vi "FindVertexOrder.vi"(5 "order":T1(ring)=enum."reverse postorder", 9 "DAG in":refnum<class "DAG.lvclass">) -> (4 "vertices":i32[](array[numeric]))   [LabVIEW 2014, in "Raspberry Pi Compatible Compiler for LabVIEW.lvlib" / "DAG.lvclass"]
uses:
  DAG.lvclass
  TypeDefs/TraversalEnum.ctl
  DAG.lvclass/DAG.ctl
  Raspberry Pi Compatible Compiler for LabVIEW.lvlib
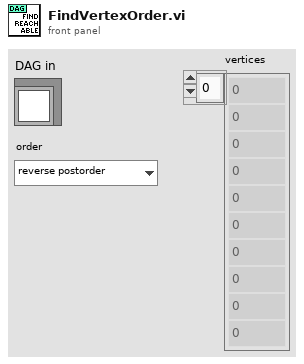
[diagram p1: front panel]
types:
  T1 = enum16{"preorder", "postorder", "reverse postorder"}
  T2 = typedef "Raspberry Pi Compatible Compiler for LabVIEW.lvlib/TraversalEnum.ctl" = enum16{"dfs", "pre-enqueue", "post-enqueue"}
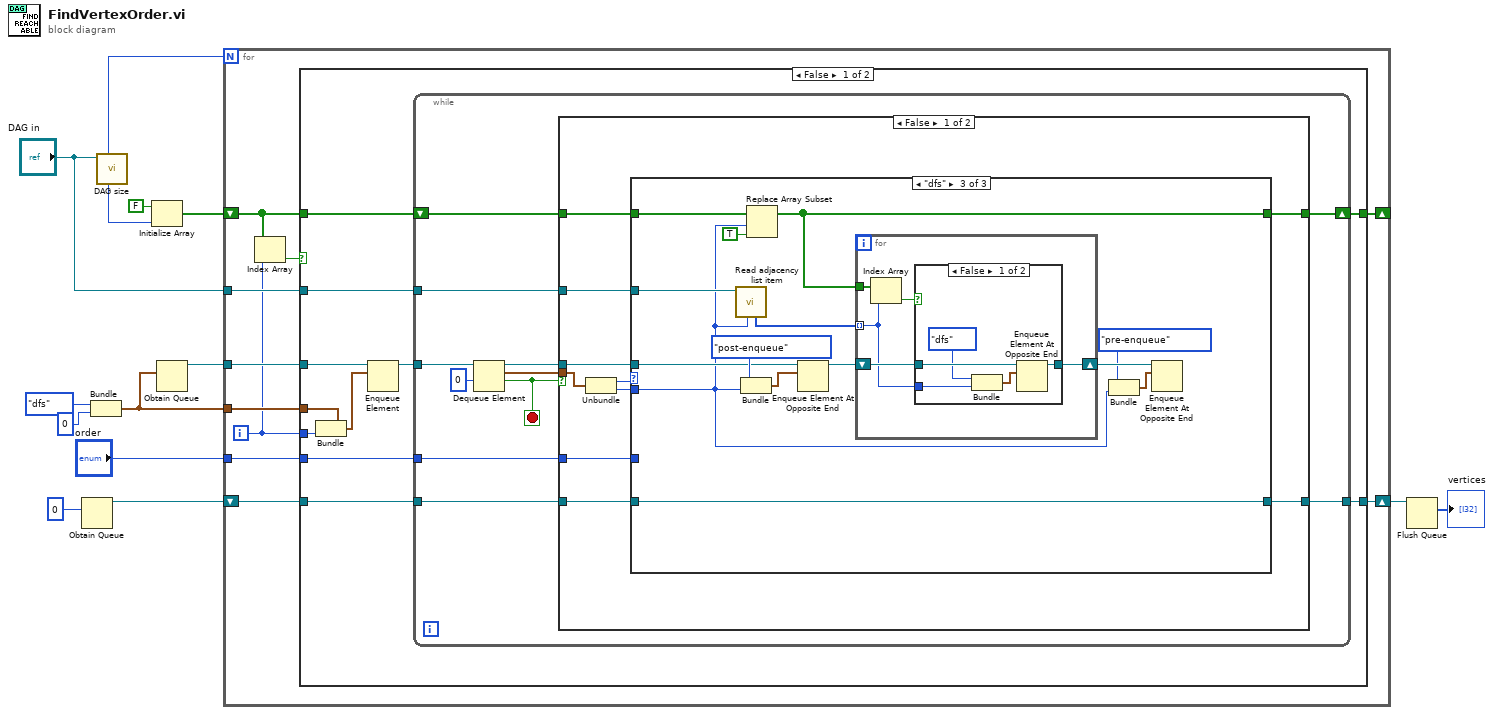
[diagram p0: block diagram]
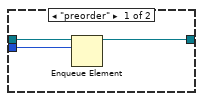
[diagram p3: hidden frame]
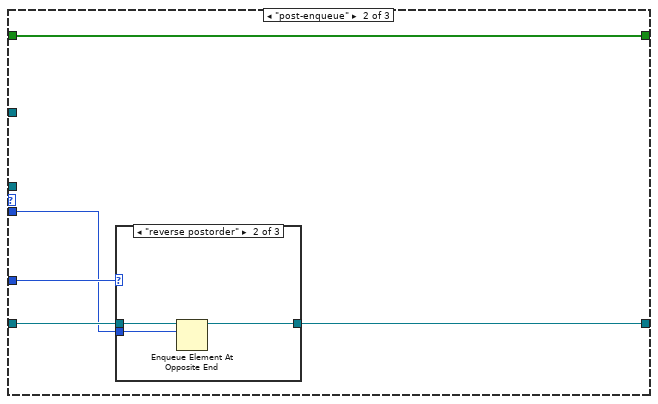
[diagram p4: hidden frame]
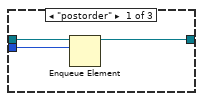
[diagram p5: hidden frame]
diagram:
  n1 = Obtain Queue(element data type=0 ("element")) -> (queue out=w5:refnum<queue>)  [unwired: 4 in, 2 out]
  n2 = Bundle(TraversalEnum."dfs", "element"=0) -> (w2:cluster{T2, "element":i32})  [unwired: 1 in]
  n3 = call "DAG size.vi"("DAG in"="DAG in") -> ("vertices"=w1:i32)  [unwired: 6 in, 2 out]
  n4 = Initialize Array(FALSE, w1) -> (w9:bool[])
  n5 = Obtain Queue(element data type=w2) -> (queue out=w10:refnum<queue>)  [unwired: 4 in, 2 out]
  n6 = for {
    N: w1 -> [_]
    tunnel: "DAG in" -> [w23]
    tunnel: w10 -> [w22]
    tunnel: "order" -> [w20]
    tunnel: w2 -> [w18]
    shift-right: [w17] -> _
    shift-left: w9 -> [w16]
    shift-right: [w19] -> w3
    shift-left: w5 -> [w21]
    i -> [w15]
    n7 = Index Array(array=w16, index=w15) -> (element=w14:bool)
    n8 = case shown="False" w14 {
      tunnel: w23 -> [w34 _]
      tunnel: w22 -> [w33 _]
      tunnel: w21 -> [w31 w104]
      tunnel: w20 -> [w30 _]
      tunnel: [w29 w104] -> w19
      tunnel: w18 -> [w28 _]
      tunnel: [w26 w105] -> w17
      tunnel: w16 -> [w25 w105]
      tunnel: w15 -> [w24 _]
      frame False {
        n9 = Bundle(cluster=w28, "element"=w24) -> (w27:cluster{T2, "element":i32})  [unwired: 1 in]
        n10 = Enqueue Element(queue=w33, element=w27) -> (queue out=w32:refnum<queue>)  [unwired: 2 in, 2 out]
        n11 = while {
          shift-right: [w42] -> w26
          shift-left: w25 -> [w41]
          tunnel: w32 -> [w45]
          tunnel: w34 -> [w40]
          tunnel: w31 -> [w37]
          tunnel: [w36] -> w29
          tunnel: w30 -> [w35]
          stop <- w43 stop-if-true
          n12 = Dequeue Element(queue=w45, timeout in ms (-1)=0) -> (queue out=w39:refnum<queue>, element=w38:cluster{T2, "element":i32}, timed out?=w43:bool)  [unwired: 1 in, 1 out]
          n13 = case shown="False" w43 {
            tunnel: w39 -> [w55 _]
            tunnel: [w53 w103] -> w42
            tunnel: w41 -> [w46 w103]
            tunnel: w38 -> [w52 _]
            tunnel: w40 -> [w54 _]
            tunnel: w37 -> [w50 w102]
            tunnel: [w49 w102] -> w36
            tunnel: w35 -> [w48 _]
            frame False {
              n14 = Unbundle(w52) -> (w51:T2, "element"=w47:i32)
              n15 = case shown="\"dfs\"" w51 {
                tunnel: w46 -> [w56 w65 w87]
                tunnel: w55 -> [_ _ w80]
                tunnel: w54 -> [_ _ w90]
                tunnel: [w56 w65 w89] -> w53
                tunnel: w47 -> [w58 w67 w78]
                tunnel: w50 -> [w59 w68 w88]
                tunnel: [w57 w66 w88] -> w49
                tunnel: w48 -> [w60 w69 _]
                frame "pre-enqueue" {
                  n16 = case shown="Default" w60 {
                    tunnel: w59 -> [w63 w64]
                    tunnel: w58 -> [w62 _]
                    tunnel: [w61 w64] -> w57
                    frame "preorder" {
                      n17 = Enqueue Element(queue=w63, element=w62) -> (queue out=w61:refnum<queue>)  [unwired: 2 in, 2 out]
                    }
                    frame Default {
                    }
                  }
                }
                frame "post-enqueue" {
                  n18 = case shown="\"reverse postorder\"" w69 {
                    tunnel: w68 -> [w72 w75 w76]
                    tunnel: w67 -> [w71 w73 _]
                    tunnel: [w70 w74 w76] -> w66
                    frame "postorder" {
                      n19 = Enqueue Element(queue=w72, element=w71) -> (queue out=w70:refnum<queue>)  [unwired: 2 in, 2 out]
                    }
                    frame "reverse postorder" {
                      n20 = Enqueue Element At Opposite End(queue=w75, element=w73) -> (queue out=w74:refnum<queue>)  [unwired: 2 in, 2 out]
                    }
                    frame Default {
                    }
                  }
                }
                frame "dfs" {
                  n21 = call "Read adjacency list item.vi"("vertex"=w78, "DAG in"=w90) -> ("edge list"=w77:i32[])  [unwired: 6 in, 1 out]
                  n22 = Bundle(TraversalEnum."post-enqueue", "element"=w78) -> (w81:cluster{T2, "element":i32})  [unwired: 1 in]
                  n23 = Replace Array Subset(array=w87, new element=TRUE ("new element/subarray"), index=w78) -> (w89:bool[])
                  n24 = Enqueue Element At Opposite End(queue=w80, element=w81) -> (queue out=w79:refnum<queue>)  [unwired: 2 in, 2 out]
                  n25 = for {
                    tunnel: w77 -> [w91] mode=indexing
                    tunnel: w89 -> [w94]
                    shift-right: [w92] -> w85
                    shift-left: w79 -> [w95]
                    n26 = Index Array(array=w94, index=w91) -> (element=w93:bool)
                    n27 = case shown="False" w93 {
                      tunnel: w95 -> [w100 w101]
                      tunnel: w91 -> [w99 _]
                      tunnel: [w97 w101] -> w92
                      frame False {
                        n28 = Bundle(TraversalEnum."dfs", "end vertex"=w99) -> (w98:cluster{T2, "end vertex":i32})  [unwired: 1 in]
                        n29 = Enqueue Element At Opposite End(queue=w100, element=w98) -> (queue out=w97:refnum<queue>)  [unwired: 2 in, 2 out]
                      }
                      frame True {
                      }
                    }
                  }
                  n30 = Bundle(TraversalEnum."pre-enqueue", "element"=w78) -> (w84:cluster{T2, "element":i32})  [unwired: 1 in]
                  n31 = Enqueue Element At Opposite End(queue=w85, element=w84) -> ()  [unwired: 2 in, 3 out]
                }
              }
            }
            frame True {
            }
          }
        }
      }
      frame True {
      }
    }
  }
  n32 = Flush Queue(queue=w3) -> (remaining elements=→"vertices":i32[])  [unwired: 1 in, 2 out]
